vi "HEWH Find Start Stop Draw Indexes.vi"(8 "error in (no error)":errorcluster, 10 "End of First Draw":i32, 11 "Full Data Output in":string[][](array[string])) -> (0 "error out":errorcluster, 2 "Draw End Index":i32, 3 "Draw Start Index":i32)   [LabVIEW 2016]
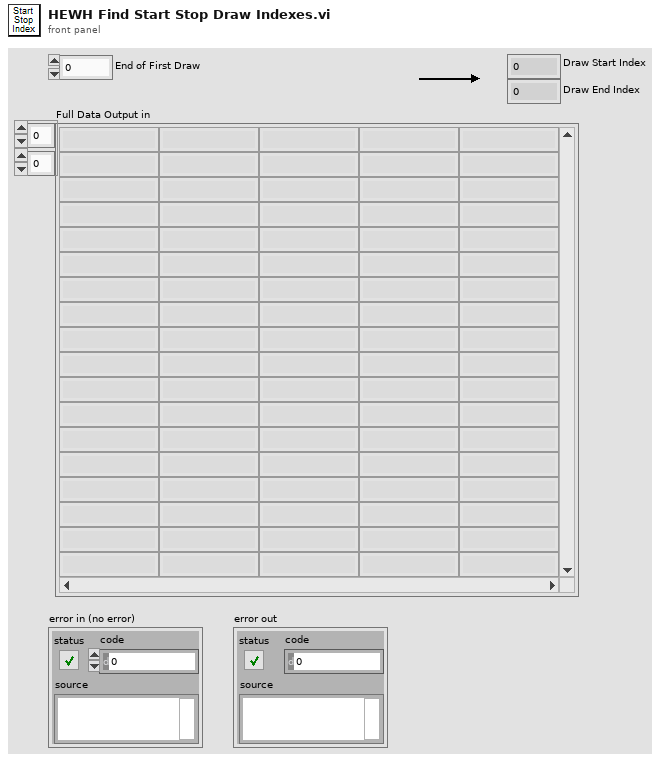
[diagram p1: front panel]
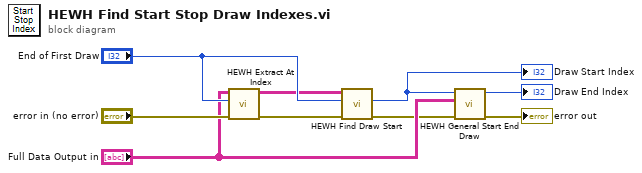
[diagram p0: block diagram]
diagram:
  n1 = call "HEWH Extract At Index.vi"("Error In"="error in (no error)", "Test Start Index in"="End of First Draw", "all rows in"="Full Data Output in") -> ("Error Out"=w7:errorcluster, "Array"=w6:string[][])  [unwired: 6 in, 1 out]
  n2 = call "HEWH Find Draw Start.vi"("Error In"=w7, "End of First Draw"="End of First Draw", "Array"=w6) -> ("Error Out"=w2:errorcluster, "Draw Start"=w4:i32)  [unwired: 7 in]
  "Draw Start Index" <- w4
  n3 = call "HEWH General Start End Draw.vi"("error in (no error)"=w2, "Full Data Input"="Full Data Output in", "Start Index"=w4) -> ("error out"=→"error out":errorcluster, "End Index"=→"Draw End Index":i32)  [unwired: 7 in]
